vi "配置文件.vi"() -> (0 "错误输出":errorcluster, 3 "配置文件线程":cluster{"配置文件":refnum<queue>})   [LabVIEW 2021]
uses:
  QueueLib/QueueLib.lvlib
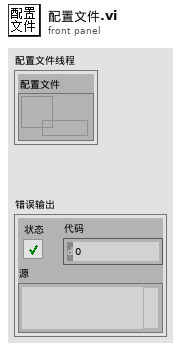
[diagram p1: front panel]
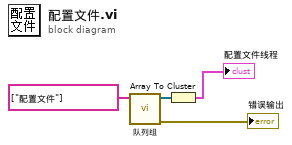
[diagram p0: block diagram]
diagram:
  n1 = call "队列组.vi"("队列名称"=string[] ["配置文件"]) -> ("错误输出"=→"错误输出":errorcluster, "队列组"=w2:refnum<queue>[])  [unwired: 9 in]
  n2 = Array To Cluster(array=w2) -> (cluster=→"配置文件线程":cluster{"队列组[0]":refnum<queue>})
